vi "FGV reentrant.vi"(8 "Error In":errorcluster, 9 "Data in":variant, 10 "Attribute Name":string, 11 "Action (read)":T1=enum."read") -> (0 "Error Out":errorcluster, 1 "Data out":variant, 2 "Success":bool, 4 "Attribute Names":string[](array[string]), 6 "Attribute Values":variant[](array[variant]))   [LabVIEW 2015, in "CS++Base.lvlib"]
doc: "This is a reentrant FGV using variant attributes to store data. The lookup time is O(log(n)).\n\n<B>Attention:</B> This FGV is intentionally set to reentrant. It must be wrapped into a non-reentrant VI for a specific database."
uses:
  CS++Base.lvlib
  FGV Action.ctl
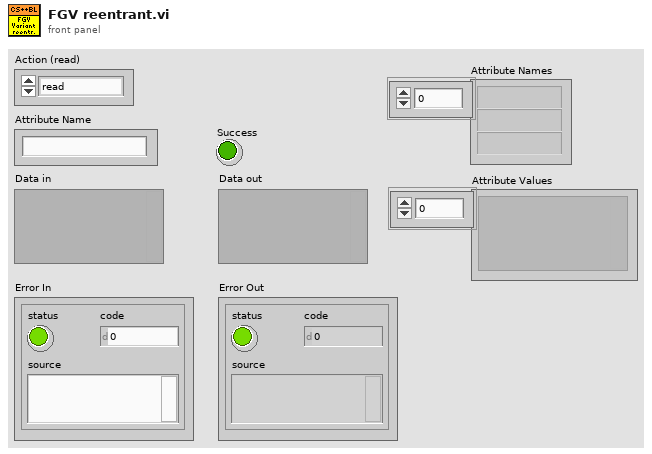
[diagram p1: front panel]
types:
  T1 = typedef "CS++Base.lvlib/FGV Action.ctl" = enum16{"add", "replace", "read", "remove", "reset", "get attributes"}
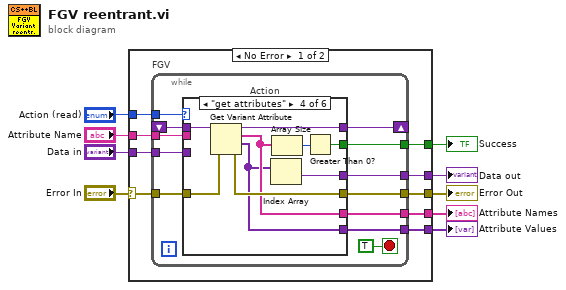
[diagram p0: block diagram]
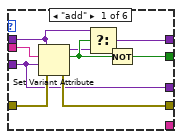
[diagram p2: hidden frame]
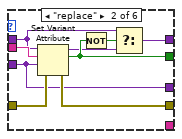
[diagram p3: hidden frame]
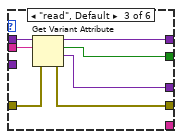
[diagram p4: hidden frame]
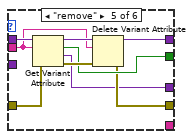
[diagram p5: hidden frame]
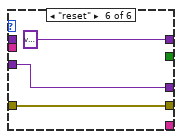
[diagram p6: hidden frame]
diagram:
  n1 = case shown="No Error" "Error In" {
    selector: "Error In" -> [w15 w77]
    tunnel: "Action (read)" -> [w18 _]
    tunnel: "Attribute Name" -> [w17 _]
    tunnel: "Data in" -> [w16 w78]
    tunnel: [w14 w78] -> w5
    tunnel: [w13 w77] -> w4
    tunnel: [w12 _] -> w3
    tunnel: [w11 _] -> w2
    tunnel: [w10 _] -> w1
    frame No Error {
      n2 = while "FGV" {
        tunnel: w18 -> [w29]
        shift-right: [w28] -> _
        shift-left: _ -> [w27]
        tunnel: w17 -> [w26]
        tunnel: w16 -> [w25]
        tunnel: w15 -> [w24]
        tunnel: [w23] -> w14
        tunnel: [w22] -> w13
        tunnel: [w21] -> w12
        tunnel: [w20] -> w11
        tunnel: [w19] -> w10
        stop <- TRUE stop-if-true
        n3 = case "Action" shown="\"get attributes\"" w29 {
          tunnel: [w32 w42 w52 w63 w73 variant] -> w28
          tunnel: w27 -> [w34 w43 w55 w64 w71 _]
          tunnel: w26 -> [w39 w48 w54 _ w69 _]
          tunnel: w25 -> [w36 w45 _ _ _ w74]
          tunnel: w24 -> [w38 w47 w53 w62 w67 w75]
          tunnel: [w36 w45 w51 w57 w65 w74] -> w23
          tunnel: [w37 w46 w50 w61 w66 w75] -> w22
          tunnel: [w31 w44 w49 w56 w68 _] -> w21
          tunnel: [_ _ _ w60 _ _] -> w20
          tunnel: [_ _ _ w58 _ _] -> w19
          frame "add" {
            n4 = Set Variant Attribute(Variant=w34, name=w39, value=w36, error in=w38) -> (Variant out=w33:variant, replaced=w35:bool, error out=w37:errorcluster)
            n5 = Select(t=w34, s=w35, f=w33) -> (s? t:f=w32:variant)
            n6 = Not(x=w35) -> (.not. x?=w31:bool)
          }
          frame "replace" {
            n7 = Set Variant Attribute(Variant=w43, name=w48, value=w45, error in=w47) -> (Variant out=w41:variant, replaced=w44:bool, error out=w46:errorcluster)
            n8 = Not(x=w44) -> (.not. x?=w40:bool)
            n9 = Select(t=w43, s=w40, f=w41) -> (s? t:f=w42:variant)
          }
          frame "read", Default {
            n10 = Get Variant Attribute(Variant=w55, name=w54, error in=w53) -> (duplicate Variant=w52:variant, found=w49:bool, value=w51:variant, error out=w50:errorcluster)  [unwired: 1 in]
          }
          frame "get attributes" {
            n11 = Get Variant Attribute(Variant=w64, error in=w62) -> (duplicate Variant=w63:variant, names=w60:string[], values=w58:variant[], error out=w61:errorcluster)  [unwired: 2 in]
            n12 = Index Array(array=w58) -> (element=w57:variant)  [unwired: 1 in]
            n13 = Array Size(array=w60) -> (size(s)=w59:i32)
            n14 = Greater Than 0?(x=w59) -> (x > 0?=w56:bool)
          }
          frame "remove" {
            n15 = Get Variant Attribute(Variant=w71, name=w69, error in=w67) -> (duplicate Variant=w70:variant, found=w68:bool, value=w65:variant, error out=w72:errorcluster)  [unwired: 1 in]
            n16 = Delete Variant Attribute(4:w72, 6:w69, 7:w70) -> (0:w66:errorcluster, 3:w73:variant)  [unwired: 1 out]
          }
          frame "reset" {
          }
        }
      }
    }
    frame Error {
    }
  }
  "Error Out" <- w4
  "Data out" <- w5
  "Success" <- w3
  "Attribute Values" <- w1
  "Attribute Names" <- w2
